vi "a4i.vi"() -> ()   [LabVIEW 2019]
uses:
  <vilib>/addons/Control Design/_Model Construction/Data Typedefs.llb/CD MIMO Time Response Data.ctl
  <vilib>/addons/Control Design/_Model Construction/Data Typedefs.llb/CD Plot Types Enum.ctl
  <vilib>/addons/Control Design/_Model Construction/Special Model Creation.llb/Special Model Creation SubVI/CD Create 2nd Order Model.vi
  <vilib>/addons/Control Design/_Time Response Analysis/Time Response.llb/Time Response subVI/cd_Step Response (Transfer Function).vi
  <vilib>/addons/Control Design/_Utility/Model Viewer.llb/Model Viewer SubVI/cd_Draw Transfer Function Equation (TF).vi
  <vilib>/addons/Control Design/_Utility/NI_CD_Model Viewer.lvlib
  <vilib>/addons/Control Design/_Model Construction/NI_CD_Special Model Creation.lvlib
  <vilib>/addons/Control Design/_Time Response Analysis/NI_CD_Time Response.lvlib
  <vilib>/addons/Control Design/_Model Construction/NI_LinSys_Data Typedefs.lvlib
panel:
  out "Damping Ratio":dbl
  out "Natural Frequency (rad/s)":dbl
  out "Static Gain":dbl=1.0
  out "Step Response Graph":cluster{"time":dbl[], dbl[]}[](graph)
  out "Step Response Data":T1={"Time"=[], "Outputs Data"=[], "States Data"=[], "plot type"=enum."step"} {"States Data" format="%#.6g"; "Outputs Data" format="%#.6g"; "Time" format="%#.6g"}
  out "Equation":picture
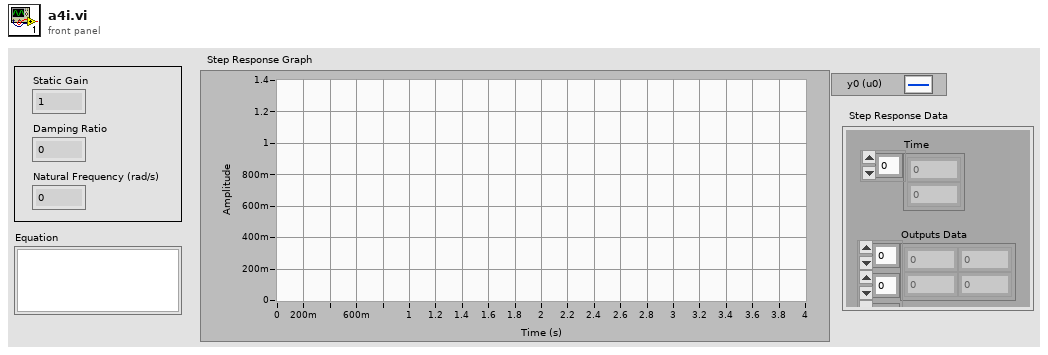
[diagram p1: front panel]
types:
  T1 = typedef "NI_LinSys_Data Typedefs.lvlib/CD MIMO Time Response Data.ctl" = cluster{"Time":dbl[], "Outputs Data":dbl[][][], "States Data":dbl[][][], "plot type":T2}
  T2 = typedef "NI_LinSys_Data Typedefs.lvlib/CD Plot Types Enum.ctl" = enum16{"bode-magnitude", "bode-phase", "nichols", "nyquist", "singular values", "step", "impulse", "initial", "simulation", "nyquist with separation"}
  T3 = typedef "NI_LinSys_Model Typedefs.lvlib/CD Transfer Function Model (MIMO).ctl" = cluster{"properties":T4, "transfer function(s)":T5[][]}
  T4 = typedef "NI_LinSys_Model Typedefs.lvlib/CD General Elements.ctl" = cluster{"Model name":string, "Input names":string[], "Output names":string[], "Input Delays":dbl[], "Output Delays":dbl[], "Sampling Time":dbl, "Notes":string}
  T5 = typedef "NI_LinSys_Model Typedefs.lvlib/CD Transfer Function Model (SISO).ctl" = cluster{"Numerator":dbl[], "Denominator":dbl[], "delay":dbl}
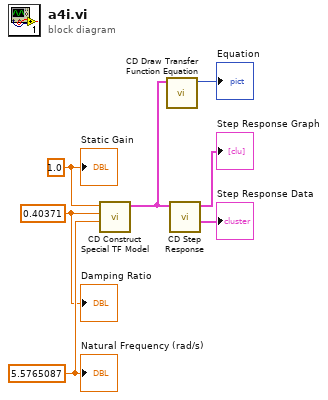
[diagram p0: block diagram]
diagram:
  w1 = 0.40371 ("Damping Ratio")
  w2 = 5.5765087 ("Natural Frequency (rad/s)")
  w3 = 1.0 ("Static Gain")
  n1 = call-poly <vilib>:"CD Construct Special TF Model.vi"("Natural Frequency (rad/s)"=w2, "Damping Ratio"=w1, "Static Gain"=w3) -> ("Transfer Function Model"=w4:T3)  [unwired: 7 in, 1 out]
  n2 = call-poly <vilib>:"CD Draw Transfer Function Equation.vi"("Transfer Function Model"=w4) -> ("Equation"=→"Equation":picture)  [unwired: 8 in, 2 out]
  n3 = call-poly <vilib>:"CD Step Response.vi"("Transfer Function Model"=w4) -> ("Step Response Data"=→"Step Response Data":T1, "Step Response Graph"=→"Step Response Graph":cluster{"time":dbl[], dbl[]}[])  [unwired: 8 in, 1 out]
  "Static Gain" <- w3
  "Natural Frequency (rad/s)" <- w2
  "Damping Ratio" <- w1
